vi "alertmessage.vi"(2 "error in (no error)":errorcluster, 3 "reply content":string) -> (0 "error out":errorcluster, 1 "body":string)   [LabVIEW 2016]
doc: "Format the message to follow dripline standard"
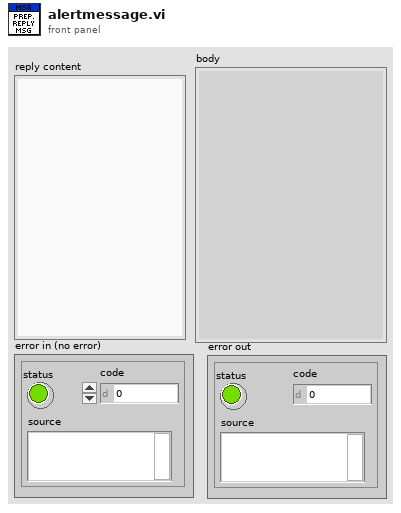
[diagram p1: front panel]
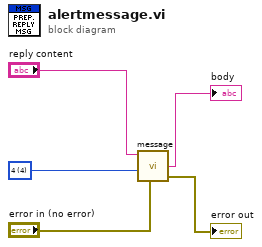
[diagram p0: block diagram]
diagram:
  w4 = 4 items=["2"=2, "3"=3, "4"=4] ("msgtype")
  n1 = call "message.vi"("input json string"="reply content", "msgtype"=w4, "error in (no error)"="error in (no error)") -> ("body"=→"body":string, "error out"=→"error out":errorcluster)  [unwired: 4 in]
